vi "ODE Linear System Symbolic.vi"(2 "X0 (start value)":dbl[](array[numeric]) format="%.2f", 3 "A (matrix of coefficients)":dbl[][](array[numeric]) format="%.2f") -> (0 "error":i32, 1 "formula":string=" ")   [LabVIEW 2010, in "NI_Gmath.lvlib"]
doc: "Solves an n-dimension linear system of differential equations with a given start condition. The solution is based on the determination of the eigenvalues and eigenvectors of the underlying matrix. The solution is given in symbolic form."
uses:
  NI_Gmath.lvlib
  Real Eigenvalues and Vectors.vi
  Complex Matrix Rank.vi
  Absolute Value - CM.vi
  Complex Inverse Matrix.vi
  Complex A x Vector.vi
  NI_AALBase.lvlib
  NI_AALPro.lvlib
  NI_Matrix.lvlib
panel:
  # "Example:\n\n A: ((1.0,2.0),(-2.3,1.1)) \n X0: 1.0 and 2.4"
  # "dX(t)/dt = AX(t)\nX(0) = X0"
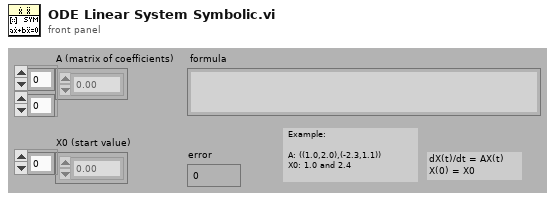
[diagram p1: front panel]
types:
  T1 = typedef "NI_Matrix.lvlib/ComplexMatrix.ctl" = cdb[][]
  T2 = typedef "NI_Matrix.lvlib/RealMatrix.ctl" = dbl[][]
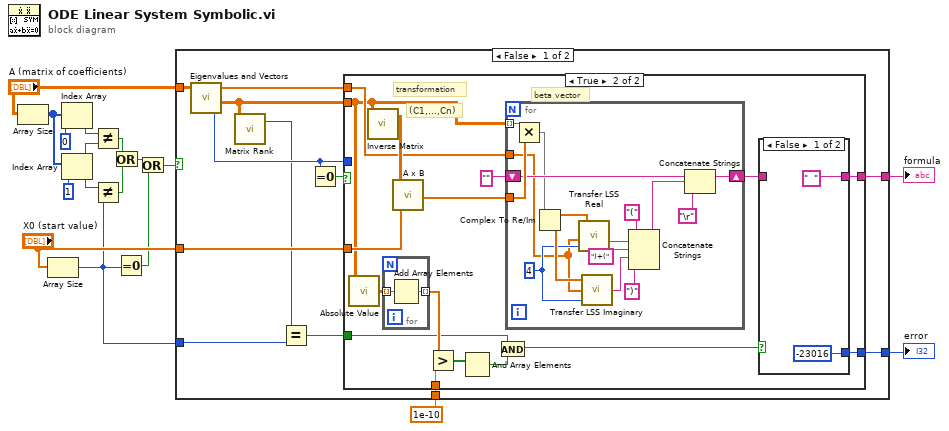
[diagram p0: block diagram]
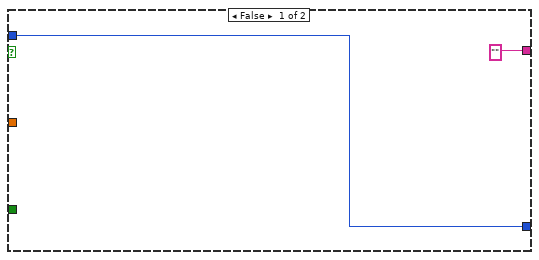
[diagram p2: hidden frame]
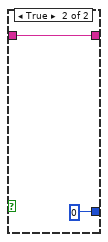
[diagram p3: hidden frame]
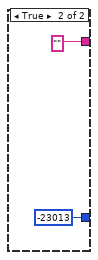
[diagram p4: hidden frame]
diagram:
  n1 = Array Size(array="A (matrix of coefficients)") -> (size(s)=w12:i32[])
  n2 = Array Size(array="X0 (start value)") -> (size(s)=w1:i32)
  n3 = Index Array(array=w12, index=0) -> (element=w14:i32)
  n4 = Index Array(array=w12, index=1) -> (element=w13:i32)
  n5 = Not Equal?(x=w14, y=w13) -> (x != y?=w11:bool)
  n6 = Not Equal?(x=w13, y=w1) -> (x != y?=w10:bool)
  n7 = Or(x=w11, y=w10) -> (x .or. y?=w6:bool)
  n8 = Equal To 0?(x=w1) -> (x = 0?=w5:bool)
  n9 = Or(x=w6, y=w5) -> (x .or. y?=w4:bool)
  n10 = case shown="False" w4 {
    tunnel: [w28 -23013] -> w9
    tunnel: "A (matrix of coefficients)" -> [w23 _]
    tunnel: "X0 (start value)" -> [w27 _]
    tunnel: [w24 ""] -> w2
    tunnel: 1e-10 -> [w22 _]
    tunnel: w1 -> [w18 _]
    frame False {
      n11 = call-poly "Eigenvalues and Vectors.vi"("Input Matrix"=w23) -> ("error"=w26:i32, "Eigenvectors"=w20:T1, "Eigenvalues"=w21:cdb[])  [unwired: 2 in]
      n12 = call-poly "Matrix Rank.vi"("Input Matrix"=w20) -> ("rank"=w19:i32)  [unwired: 1 in, 1 out]
      n13 = Equal?(x=w19, y=w18) -> (x = y?=w17:bool)
      n14 = Equal To 0?(x=w26) -> (x = 0?=w25:bool)
      n15 = case shown="True" w25 {
        tunnel: ["" w40] -> w24
        tunnel: w20 -> [_ w33]
        tunnel: w21 -> [_ w43]
        tunnel: w27 -> [_ w46]
        tunnel: [w30 w39] -> w28
        tunnel: w26 -> [w30 _]
        tunnel: w22 -> [_ w37]
        tunnel: w17 -> [_ w31]
        frame False {
        }
        frame True {
          # "transformation"
          # "beta vector"
          # "(C1,...,Cn)"
          n16 = call-poly "Absolute Value.vi"("Complex Matrix A"=w33) -> ("|A|"=w38:T2)
          n17 = call-poly "Inverse Matrix.vi"("Input Matrix"=w33) -> ("Inverse Matrix"=w45:T1)  [unwired: 1 in, 1 out]
          n18 = for {
            tunnel: w38 -> [w48] mode=indexing
            tunnel: [w47] -> w32 mode=indexing
            n19 = Add Array Elements(numeric array=w48) -> (sum=w47:dbl)
          }
          n20 = call-poly "A x B.vi"("Vector"=w46, "A"=w45) -> ("A x Vector"=w44:cdb[])  [unwired: 1 out]
          n21 = Greater?(x=w32, y=w37) -> (0:w36:bool[])
          n22 = And Array Elements(Boolean array=w36) -> (logical AND=w35:bool)
          n23 = And(x=w31, y=w35) -> (x .and. y?=w34:bool)
          n24 = for {
            tunnel: w44 -> [w67]
            tunnel: w33 -> [w68] mode=indexing
            tunnel: w43 -> [w54]
            shift-right: [w66] -> w41
            shift-left: "" -> [w65]
            w55 = u32 4
            n25 = Multiply(x=w68, y=w67) -> (x*y=w53:cdb[])
            n26 = Complex To Re/Im(x + iy=w53) -> (x=w56:dbl[], y=w57:dbl[])
            n27 = call "Transfer LSS Real.vi"("precision"=w55, "lambda"=w54, "beta"=w56) -> ("formula linear combination"=w60:string)
            n28 = call "Transfer LSS Imaginary.vi"("precision"=w55, "lambda"=w54, "beta"=w57) -> ("formula linear combination"=w62:string)
            n29 = Concatenate Strings("(", w60, ")+(", w62, ")") -> (w58:string)
            n30 = Concatenate Strings(w65, w58, "\r") -> (w66:string)
          }
          n31 = case shown="False" w34 {
            tunnel: w41 -> [_ w52]
            tunnel: ["  " w52] -> w40
            tunnel: [-23016 0] -> w39
            frame False {
            }
            frame True {
            }
          }
        }
      }
    }
    frame True {
    }
  }
  "error" <- w9
  "formula" <- w2
